vi "App_Monitor.vi"() -> ()   [LabVIEW 2015, in "Application 2.lvlib"]
uses:
  Application 2.lvlib
  Data Def/App_Subpanel Name.ctl
  Data Def/App_User Event Data.ctl
  Data Def/App_Tips Data.ctl
panel:
  in  "Live Mode":bool=TRUE
  out "Result":string caption="String"
  in  "Update":bool
  out "Electrocardiography":waveform(dbl)(graph) caption="Waveform Graph"
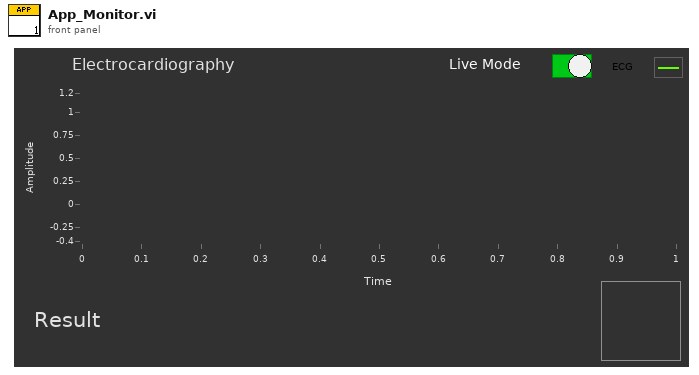
[diagram p1: front panel]
types:
  T1 = typedef "Application 2.lvlib/App_Tips Data.ctl" = cluster{"Tips":string, "BG Color":u32}
  T2 = typedef "Application 2.lvlib/App_User Event Data.ctl" = cluster{"Command":string, "Data":variant}
  T3 = typedef "Application 2.lvlib/App_Subpanel Name.ctl" = enum16{"Main", "Menu", "User Registering", "User Setting", "Monitor", "Traning Mode", "Query Data", "Connect Setting"}
  T4 = typedef "Update Result.ctl" = enum16{"Normal", "Abnormal", "Can't find training data"}
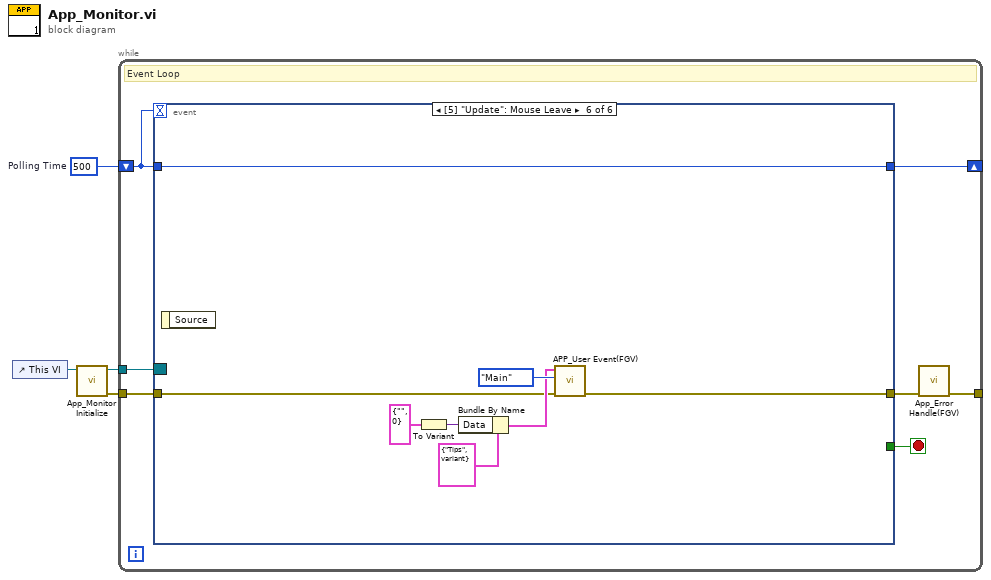
[diagram p0: block diagram]
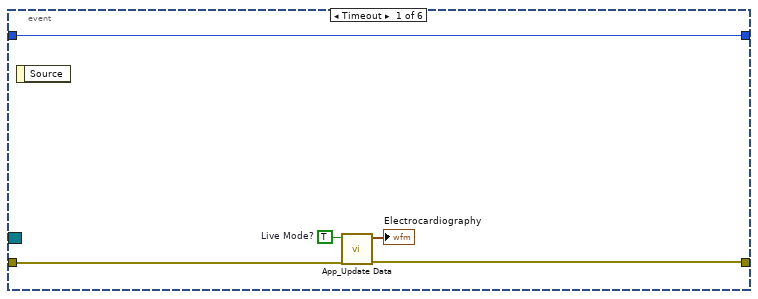
[diagram p2: hidden frame]
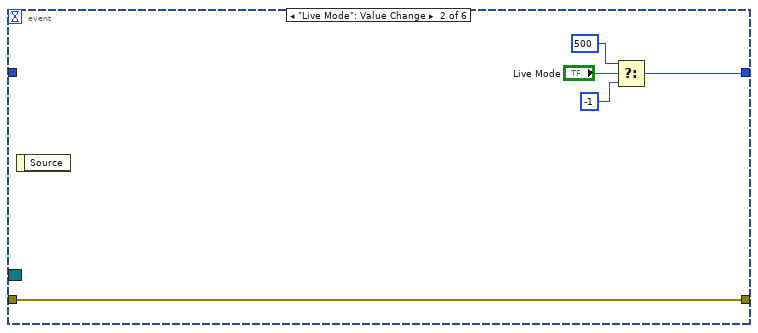
[diagram p3: hidden frame]
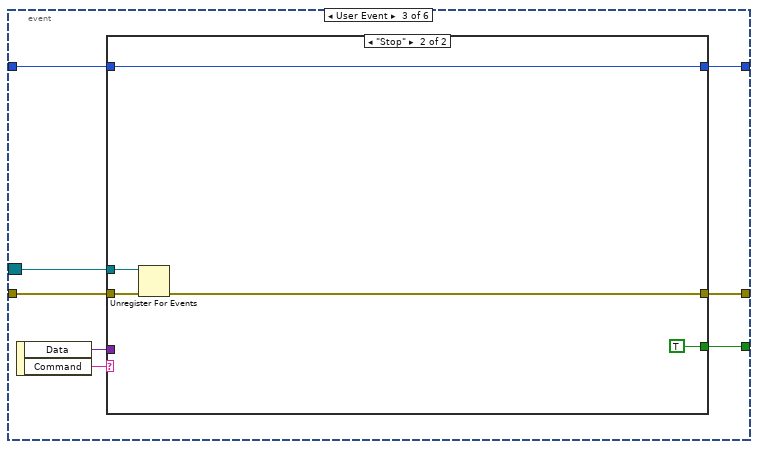
[diagram p4: hidden frame]
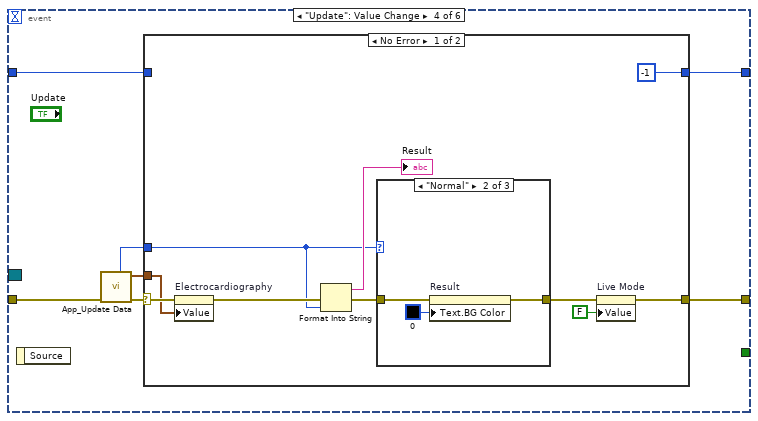
[diagram p6: hidden frame]
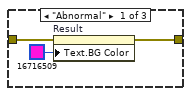
[diagram p7: hidden frame]
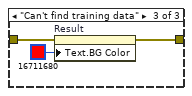
[diagram p8: hidden frame]
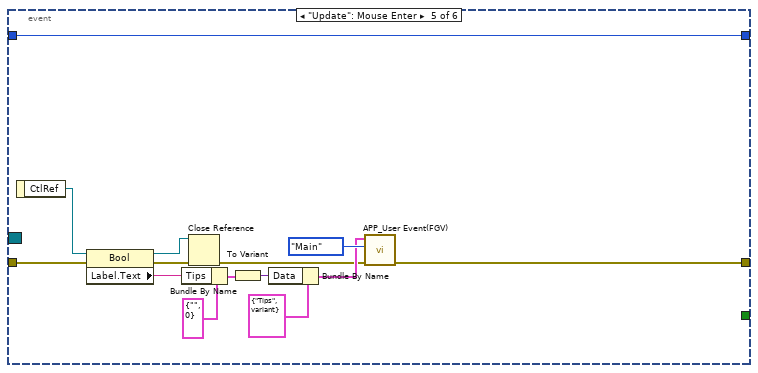
[diagram p10: hidden frame]
diagram:
  w1 = 500  # Polling Time
  n1 = control-ref of="This VI"() -> (w4:refnum<vi>)
  n2 = call "App_Monitor Initialize.vi"("VI Reference"=w4) -> ("error out"=w2:errorcluster, "Event Registration Refnum"=w3:refnum<event-registration>)  [unwired: 9 in]
  n3 = while {
    tunnel: w3 -> [w11]
    tunnel: w2 -> [w10]
    tunnel: [w7] -> _
    shift-right: [w5] -> _
    shift-left: w1 -> [w6]
    stop <- w9 stop-if-true
    # "Event Loop"
    n4 = event shown="[5] \"Update\": Mouse Leave" {
      selector: w11 -> [_ _ w26 _ _ _]
      dyn-events: _ -> [_ _ _ _ _ _]
      timeout: w6 -> [_ _ _ _ _ _]
      tunnel: w10 -> [w12 w17 w27 w43 w67 w80]
      tunnel: [w15 w17 w25 w41 w65 w79] -> w8
      tunnel: [_ _ w24 _ _ _] -> w9
      tunnel: w6 -> [w16 _ w23 w39 w78 w86]
      tunnel: [w16 w19 w22 w40 w78 w86] -> w5
      event Timeout {
        w13 = TRUE  # Live Mode?
        n5 = event-data() -> ()  [unwired: 1 in, 1 out]
        n6 = call "App_Update Data.vi"("error in"=w12, "Live Mode?(F)"=w13) -> ("error out"=w15:errorcluster, "Data"=→"Electrocardiography":waveform(dbl))  [unwired: 7 in, 1 out]
      }
      event "Live Mode": Value Change {
        n7 = event-data() -> ()  [unwired: 1 in, 1 out]
        n8 = Select(t=500, s="Live Mode", f=-1) -> (s? t:f=w19:i32)
      }
      event User Event {
        n9 = event-data() -> ("Data"=w28:variant, "Command"=w29:string)  [unwired: 1 in]
        n10 = case shown="\"Stop\"" w29 {
          tunnel: w28 -> [_ _]
          tunnel: w27 -> [w31 w36]
          tunnel: w26 -> [_ w35]
          tunnel: [w31 w34] -> w25
          tunnel: [_ TRUE] -> w24
          tunnel: w23 -> [w30 w32]
          tunnel: [w30 w32] -> w22
          frame Default {
          }
          frame "Stop" {
            n11 = Unregister For Events(event registration refnum=w35, error in=w36) -> (error out=w34:errorcluster)
          }
        }
      }
      event "Update": Value Change {
        n12 = event-data() -> ()  [unwired: 1 in, 1 out]
        n13 = call "App_Update Data.vi"("error in"=w43) -> ("error out"=w42:errorcluster, "Data"=w38:waveform(dbl), "Update Result"=w37:T4)  [unwired: 8 in]
        n14 = case shown="No Error" w42 {
          selector: w42 -> [w50 w63]
          tunnel: [w53 w63] -> w41
          tunnel: [-1 w64] -> w40
          tunnel: w39 -> [_ w64]
          tunnel: w38 -> [w49 _]
          tunnel: w37 -> [w45 _]
          frame No Error {
            n15 = property on="Electrocardiography" class="WFGraph (strict)"(error in=w50, "Value"=w49) -> (error out=w47:errorcluster)  [unwired: 1 in, 1 out]
            n16 = Format Into String(error in=w47, w45) -> (resulting string=→"Result":string, error out=w44:errorcluster)  [unwired: 2 in]
            n17 = case shown="\"Normal\"" w45 {
              tunnel: [w56 w59 w62] -> w48
              tunnel: w44 -> [w54 w57 w60]
              frame "Abnormal" {
                n18 = property on="Result" class="Str"(error in=w54, "Text.BG Color"=u32 16716509) -> (error out=w56:errorcluster)  [unwired: 1 in, 1 out]
              }
              frame "Normal" {
                n19 = property on="Result" class="Str"(error in=w57, "Text.BG Color"=u32 0) -> (error out=w59:errorcluster)  [unwired: 1 in, 1 out]
              }
              frame "Can't find training data" {
                n20 = property on="Result" class="Str"(error in=w60, "Text.BG Color"=u32 16711680) -> (error out=w62:errorcluster)  [unwired: 1 in, 1 out]
              }
            }
            n21 = property on="Live Mode" class="Bool (strict)"(error in=w48, "Value"=FALSE ("Live Mode")) -> (error out=w53:errorcluster)  [unwired: 1 in, 1 out]
          }
          frame Error {
          }
        }
      }
      event "Update": Mouse Enter {
        n22 = event-data() -> ("CtlRef"=w66:refnum<vi>)  [unwired: 1 in]
        n23 = property class="Bool"(reference=w66, error in=w67) -> (reference out=w72:refnum<vi>, error out=w73:errorcluster, "Label.Text"=w69:string)
        n24 = Bundle By Name(cluster=T1 {"Tips"="", "BG Color"=0} ("Tips Data"), "Tips"=w69) -> (w70:T1)
        n25 = Close Reference(reference=w72, error in (no error)=w73) -> (error out=w71:errorcluster)
        n26 = To Variant(anything=w70) -> (Variant=w75:variant)
        n27 = Bundle By Name(cluster=T2 {"Command"="Tips", "Data"=variant} ("User Event Data"), "Data"=w75) -> (w74:T2)
        n28 = call "APP_User Event(FGV).vi"("error in"=w71, "Subpanel Name"=App_Subpanel_Name."Main", "User Event Data"=w74) -> ("error out"=w65:errorcluster)  [unwired: 7 in, 1 out]
      }
      event "Update": Mouse Leave {
        n29 = event-data() -> ()  [unwired: 1 in, 1 out]
        n30 = To Variant(anything=T1 {"Tips"="", "BG Color"=0} ("Tips Data")) -> (Variant=w83:variant)
        n31 = Bundle By Name(cluster=T2 {"Command"="Tips", "Data"=variant} ("User Event Data"), "Data"=w83) -> (w82:T2)
        n32 = call "APP_User Event(FGV).vi"("error in"=w80, "Subpanel Name"=App_Subpanel_Name."Main", "User Event Data"=w82) -> ("error out"=w79:errorcluster)  [unwired: 7 in, 1 out]
      }
    }
    n33 = call "App_Error Handle(FGV).vi"("error in"=w8) -> ("error out"=w7:errorcluster)  [unwired: 9 in, 1 out]
  }
